vi "CallingVI.vi"() -> ()   [LabVIEW 2014]
uses:
  TimerCommands.ctl
panel:
  in  "Target Time (s)":dbl
  out "Elapsed Time":dbl
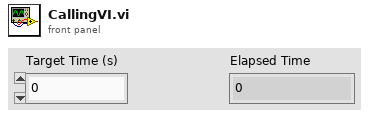
[diagram p1: front panel]
types:
  T1 = typedef "TimerCommands.ctl" = enum16{"Start", "Check Time"}
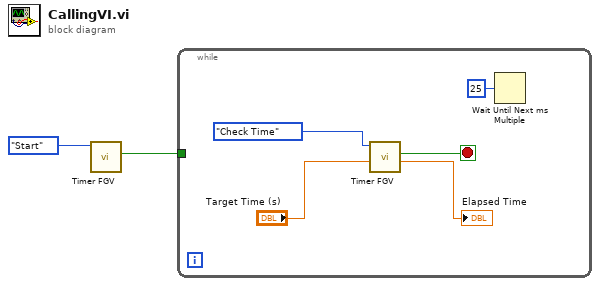
[diagram p0: block diagram]
diagram:
  n1 = call "Timer FGV.vi"("Timer Command"=TimerCommands."Start") -> ("Done?"=w2:bool)  [unwired: 9 in, 1 out]
  n2 = while {
    tunnel: w2 -> [_]
    stop <- w6 stop-if-true
    n3 = call "Timer FGV.vi"("Target Time (s)"="Target Time (s)", "Timer Command"=TimerCommands."Check Time") -> ("Elapsed Time"=→"Elapsed Time":dbl, "Done?"=w6:bool)  [unwired: 8 in]
    n4 = Wait Until Next ms Multiple(millisecond multiple=u32 25) -> ()  [unwired: 1 out]
  }
